vi "CALC_TRAN_TIME_IMP_WIDT_MIN_MAX.vi"(0 "VISA IN":refnum<visa-resource-name>, 5 "error in":errorcluster, 7 "Channel":i32, 9 "Impulse Width(sec)":dbl min=0.0 max=1.0) -> (14 "VISA Out":refnum<visa-resource-name>, 19 "error out":errorcluster)   [LabVIEW 2018, in "PNA-X.lvlib"]
doc: "CALCulate<cnum>:TRANsform:TIME:IMPulse:WIDTh <num> \n(Read-Write) Sets the impulse width for the transform window. \nSee Critical Note \nParameters \n<cnum> Channel number of the measurement. There must be a selected measurement \non that channel. If unspecified, <cnum> is set to 1. \n<num> Impulse width in seconds; Choose any number between: \n.6 / frequency span and 1.39 / frequency span \nExamples CALC:TRAN:TIME:IMP:WIDTh 10 \ncalculate2:transform:time:impulse:width 13 \nQuery Syntax CALCulate<cnum>:TRANsform:TIME:IMPulse:WIDTh? \nReturn Type Numeric \nDefault .98 / Default Span"
uses:
  PNA-X.lvlib
panel:
  out "coerced(x)":dbl
  out "x+y":dbl
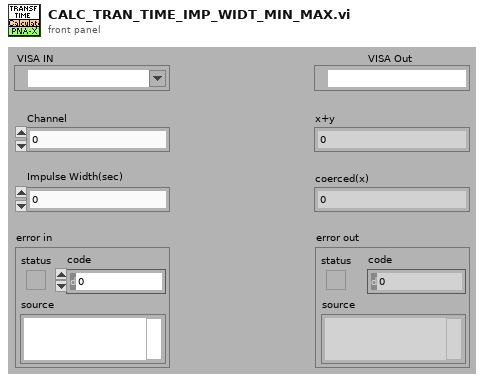
[diagram p1: front panel]
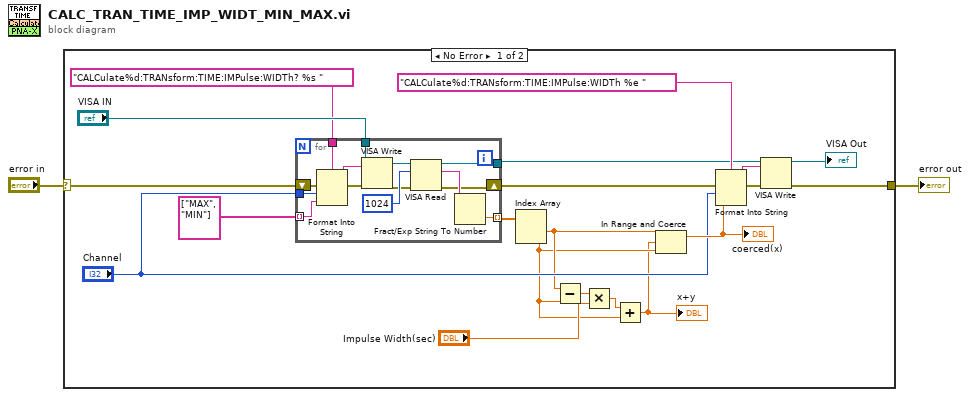
[diagram p0: block diagram]
diagram:
  n1 = case shown="No Error" "error in" {
    selector: "error in" -> [w22 w37]
    tunnel: [w9 w37] -> w1
    frame No Error {
      n2 = for {
        tunnel: "VISA IN" -> [w33]
        tunnel: "CALCulate%d:TRANsform:TIME:IMPulse:WIDTh? %s " ("Cmdline") -> [w32]
        tunnel: "Channel" -> [w31]
        tunnel: [w29] -> w11
        tunnel: string[] ["MAX", "MIN"] -> [w26] mode=indexing
        tunnel: [w24] -> w18 mode=indexing
        shift-right: [w23] -> w15
        shift-left: w22 -> [w36]
        n3 = Format Into String(format string=w32, error in=w36, w31, w26) -> (resulting string=w34:string, error out=w35:errorcluster)  [unwired: 1 in]
        n4 = VISA Write(VISA resource name=w33, write buffer=w34, error in (no error)=w35) -> (VISA resource name out=w28:refnum<visa-resource-name>, error out=w27:errorcluster)  [unwired: 1 out]
        n5 = VISA Read(VISA resource name=w28, byte count=1024, error in (no error)=w27) -> (VISA resource name out=w29:refnum<visa-resource-name>, read buffer=w25:string, error out=w23:errorcluster)  [unwired: 1 out]
        n6 = Fract/Exp String To Number(string=w25) -> (number=w24:dbl)  [unwired: 3 in, 1 out]
      }
      n7 = Index Array(array=w18) -> (element #1=w8:dbl, element #2=w4:dbl)  [unwired: 2 in]
      n8 = Subtract(x=w8, y=w4) -> (x-y=w7:dbl)
      n9 = Multiply(x=w7, y="Impulse Width(sec)") -> (x*y=w5:dbl)
      n10 = Add(x=w5, y=w4) -> (x+y=w3:dbl)
      "x+y" <- w3
      n11 = In Range and Coerce(upper limit=w8, x=w3, lower limit=w4) -> (coerced(x)=w13:dbl)  [unwired: 1 out]
      "coerced(x)" <- w13
      n12 = Format Into String(format string="CALCulate%d:TRANsform:TIME:IMPulse:WIDTh %e " ("Cmdline"), error in=w15, "Channel", w13) -> (resulting string=w16:string, error out=w17:errorcluster)  [unwired: 1 in]
      n13 = VISA Write(VISA resource name=w11, write buffer=w16, error in (no error)=w17) -> (VISA resource name out=→"VISA Out":refnum<visa-resource-name>, error out=w9:errorcluster)  [unwired: 1 out]
    }
    frame Error {
    }
  }
  "error out" <- w1
